vi "temp.vi"() -> ()   [LabVIEW 2011]
panel:
  out "字符串 2":string
  out "数字":dbl[][](array[numeric])
  in  "字符串":string="0\t30\t11.1063\n25\t38.333\t11.1187\n50\t46.667\t11.1206\n75\t55\t11.1231\n100\t63.333\t11.1276\n125\t71.667\t11.1194\n150\t80\t11.1212\n175\t88.333\t11.1185\n200\t96.667\t11.1159\n225\t105\t11.1153\n250\t113.333\t11.1188\n275\t121.667\t11.1154\n300\t130\t11.1168\n325\t138.333\t11.1172\n350\t146.667\t11.1134\n375\t155\t11.1145\n400\t163.333\t11.1154\n425\t171.667\t11.1124\n450\t180\t11.11\n475\t188.333\t11.1115\n500\t196.667\t11.1062\n525\t205\t11.1064\n550\t213.333\t11.0941\n575\t221.667\t11.095\n600\t230\t11.0884\n625\t238.333\t11.0824\n650\t246.667\t11.0654\n675\t255\t11.0513\n700\t263.333\t11.0137\n725\t271.667\t10.9618\n750\t280\t10.8607\n775\t288.333\t10.6127\n800\t296.667\t10.1264\n825\t305\t9.7119\n850\t313.333\t9.18645\n875\t321.667\t8.5292\n900\t330\t7.4518\n925\t338.333\t6.009\n950\t346.667\t4.8246\n975\t355\t4.35135\n1000\t363.333\t4.2172\n1025\t371.667\t4.1556\n1050\t380\t4.1147\n1075\t388.333\t4.08615\n1100\t396.667\t4.05485\n1125\t405\t4.0235\n1150\t413.333\t3.97715\n1175\t421.667\t3.93255\n1200\t430\t3.8579\n1225\t438.333\t3.75975\n1250\t446.667\t3.62955\n1275\t455\t3.47845\n1300\t463.333\t3.3045\n1325\t471.667\t3.1232\n1350\t480\t2.96605\n1375\t488.333\t2.82095\n1400\t496.667\t2.6908\n1425\t505\t2.59485\n1450\t513.333\t2.5324\n1475\t521.667\t2.48765\n1500\t530\t2.45995\n1525\t538.333\t2.43335\n1550\t546.667\t2.42465\n1575\t555\t2.4141\n1600\t563.333\t2.39335\n1625\t571.667\t2.38085\n1650\t580\t2.37025\n1675\t588.333\t2.3588\n1700\t596.667\t2.3499\n1725\t605\t2.34125\n1750\t613.333\t2.3317\n1775\t621.667\t2.32335\n1800\t630\t2.31785\n1825\t638.333\t2.3094\n1850\t646.667\t2.29875\n1875\t655\t2.3\n1900\t663.333\t2.29985\n1925\t671.667\t2.29685\n1950\t680\t2.29645\n1975\t688.333\t2.2954\n2000\t696.667\t2.29255\n2025\t705\t2.28145\n2050\t713.333\t2.287\n2075\t721.667\t2.2834\n2100\t730\t2.27305\n2125\t738.333\t2.27875\n2150\t746.667\t2.27465\n2175\t755\t2.2738\n2200\t763.333\t2.2764\n2225\t771.667\t2.26885\n2250\t780\t2.265\n2275\t788.333\t2.2597\n2300\t796.667\t2.26315\n2325\t805\t2.2574\n2350\t813.333\t2.2534\n2375\t821.667\t2.2464\n2400\t830\t2.2449\n2425\t838.333\t2.2434\n2450\t846.667\t2.23815\n"
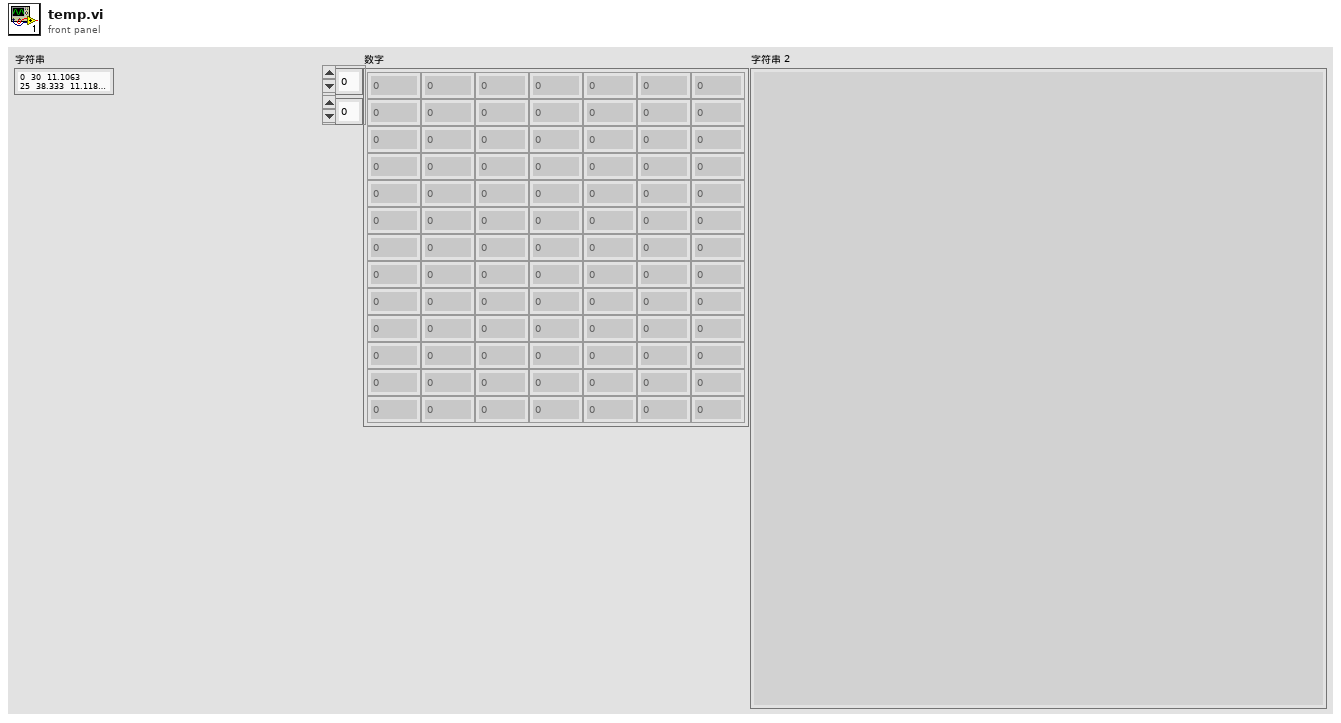
[diagram p1: front panel]
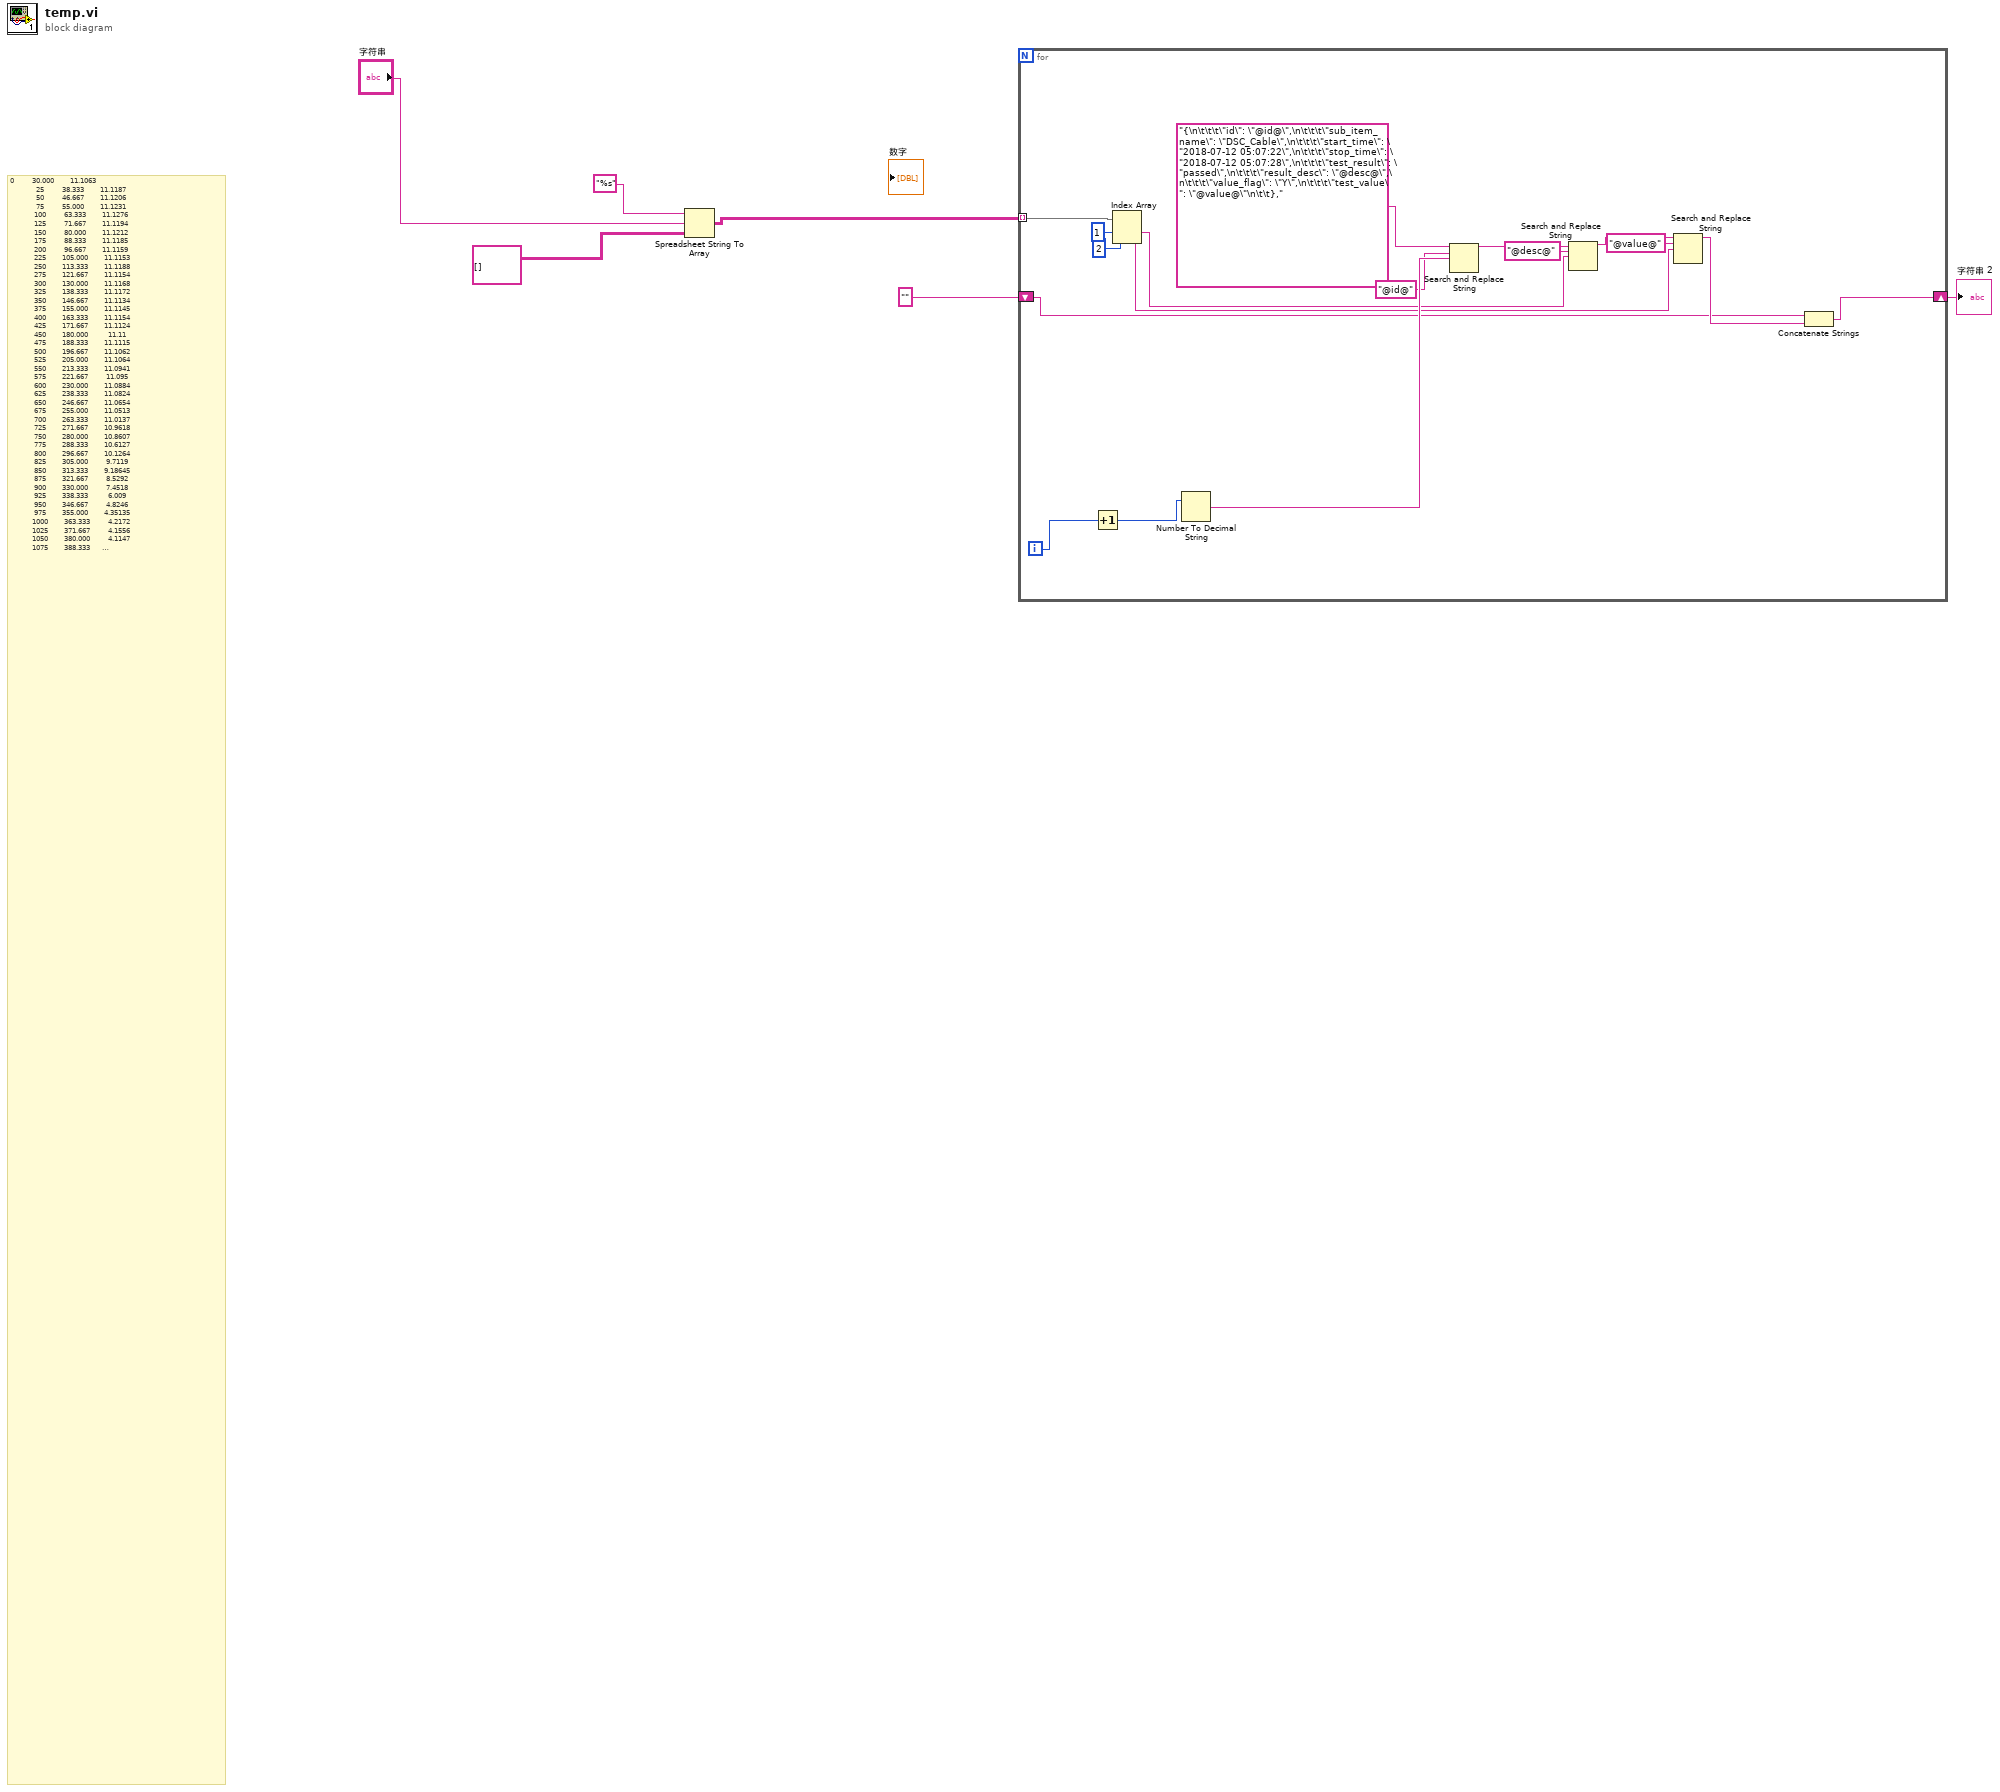
[diagram p0: block diagram]
diagram:
  # "0         30.000        11.1063\n             25         38.333        11.1187\n             50         46.667        11.1206\n             75         55.000        11.1231\n            100         63.333        11.1276\n            125         71.667        11.1194\n            150         80.000        11.1212\n            175         88.333        11.1185\n            200         96.667        11.1159\n            225        105.000        11.1153\n            250        113.333        11.1188\n            275        121.667        11.1154\n            300        130.000        11.1168\n            325        138.333        11.1172\n            350        146.667        11.1134\n            375        155.000        11.1145\n            400        163.333        11.1154\n            425        171.667        11.1124\n            450        180.000          11.11\n            475        188.333        11.1115\n            500        196.667        11.1062\n            525        205.000        11.1064\n            550        213.333        11.0941\n            575        221.667         11.095\n            600        230.000        11.0884\n            625        238.333        11.0824\n            650        246.667        11.0654\n            675        255.000        11.0513\n            700        263.333        11.0137\n            725        271.667        10.9618\n            750        280.000        10.8607\n            775        288.333        10.6127\n            800        296.667        10.1264\n            825        305.000         9.7119\n            850        313.333        9.18645\n            875        321.667         8.5292\n            900        330.000         7.4518\n            925        338.333          6.009\n            950        346.667         4.8246\n            975        355.000        4.35135\n           1000        363.333         4.2172\n           1025        371.667         4.1556\n           1050        380.000         4.1147\n           1075        388.333        4.08615\n           1100        396.667        4.05485\n           1125        405.000         4.0235\n           1150        413.333        3.97715\n           1175        421.667        3.93255\n           1200        430.000         3.8579\n           1225        438.333        3.75975\n           1250        446.667        3.62955\n           1275        455.000        3.47845\n           1300        463.333         3.3045\n           1325        471.667         3.1232\n           1350        480.000        2.96605\n           1375        488.333        2.82095\n           1400        496.667         2.6908\n           1425        505.000        2.59485\n           1450        513.333         2.5324\n           1475        521.667        2.48765\n           1500        530.000        2.45995\n           1525        538.333        2.43335\n           1550        546.667        2.42465\n           1575        555.000         2.4141\n           1600        563.333        2.39335\n           1625        571.667        2.38085\n           1650        580.000        2.37025\n           1675        588.333         2.3588\n           1700        596.667         2.3499\n           1725        605.000        2.34125\n           1750        613.333         2.3317\n           1775        621.667        2.32335\n           1800        630.000        2.31785\n           1825        638.333         2.3094\n           1850        646.667        2.29875\n           1875        655.000            2.3\n           1900        663.333        2.29985\n           1925        671.667        2.29685\n           1950        680.000        2.29645\n           1975        688.333         2.2954\n           2000        696.667        2.29255\n           2025        705.000        2.28145\n           2050        713.333          2.287\n           2075        721.667         2.2834\n           2100        730.000        2.27305\n           2125        738.333        2.27875\n           2150        746.667        2.27465\n           2175        755.000         2.2738\n           2200        763.333         2.2764\n           2225        771.667        2.26885\n           2250        780.000          2.265\n           2275        788.333         2.2597\n           2300        796.667        2.26315\n           2325        805.000         2.2574\n           2350        813.333         2.2534\n           2375        821.667         2.2464\n           2400        830.000         2.2449\n           2425        838.333         2.2434\n           2450        846.667        2.23815"
  n1 = Spreadsheet String To Array(format string="%s" ("电子表格字符串"), spreadsheet string="字符串", array type (2D Dbl)=string[][] [] ("数组类型(2D Dbl)")) -> (array=w3:string[][])  [unwired: 1 in]
  n2 = for {
    tunnel: w3 -> [w21] mode=indexing
    shift-right: [w7] -> w1
    shift-left: "" ("字符串") -> [w8]
    i -> [w19]
    n3 = Increment(x=w19) -> (x+1=w18:i32)
    n4 = Index Array(array=w21, index #1=1 ("索引"), index #2=2 ("索引")) -> (element #1=w13:string, element #2=w10:string)
    n5 = Number To Decimal String(number=w18) -> (decimal integer string=w17:string)  [unwired: 1 in]
    n6 = Search and Replace String(input string="{\n\t\t\t\"id\": \"@id@\",\n\t\t\t\"sub_item_name\": \"DSC_Cable\",\n\t\t\t\"start_time\": \"2018-07-12 05:07:22\",\n\t\t\t\"stop_time\": \"2018-07-12 05:07:28\",\n\t\t\t\"test_result\": \"passed\",\n\t\t\t\"result_desc\": \"@desc@\",\n\t\t\t\"value_flag\": \"Y\",\n\t\t\t\"test_value\": \"@value@\"\n\t\t},", search string="@id@" ("搜索字符串"), replace string=w17) -> (result string=w15:string)  [unwired: 5 in, 3 out]
    n7 = Search and Replace String(input string=w15, search string="@desc@" ("搜索字符串"), replace string=w13) -> (result string=w12:string)  [unwired: 5 in, 3 out]
    n8 = Search and Replace String(input string=w12, search string="@value@" ("搜索字符串"), replace string=w10) -> (result string=w9:string)  [unwired: 5 in, 3 out]
    n9 = Concatenate Strings(w8, w9) -> (w7:string)
  }
  "字符串 2" <- w1
